vi "File Page - Set .NET Filter.vi"(7 "Include Wfms?":bool, 8 "error in (no error)":errorcluster, 11 "Trigger Control in":T1) -> (0 "error out":errorcluster, 3 "Trigger Control out":T1)   [LabVIEW 2015, in "Waveform Data Logger System Explorer.lvlib"]
uses:
  Waveform Data Logger System Explorer.lvlib
  <vilib>/NI Veristand/UI Controls/Single Node Browser/Single Node Browser Ref.ctl
  NationalInstruments.VeriStand.SystemStorageUI
  NationalInstruments.VeriStand.SystemStorage
  <vilib>/NI VeriStand/UI Controls/Single Node Browser/NI_VS UI Single Node Browser.lvlib
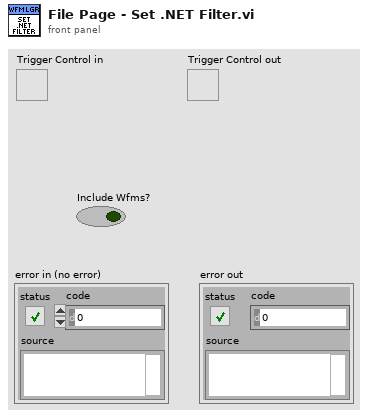
[diagram p1: front panel]
types:
  T1 = typedef "NI_VS UI Single Node Browser.lvlib/Single Node Browser Ref.ctl" = refnum<k24>
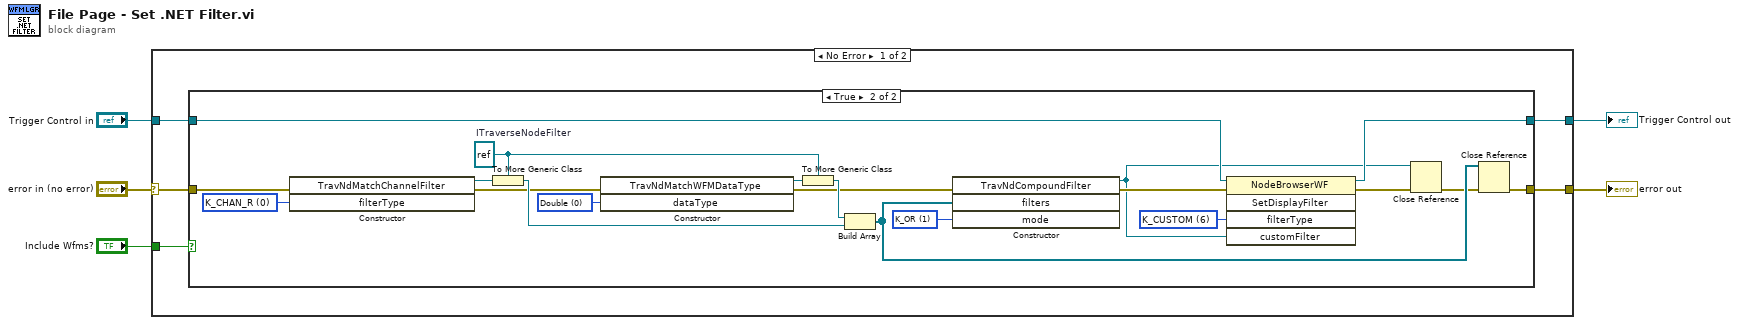
[diagram p0: block diagram]
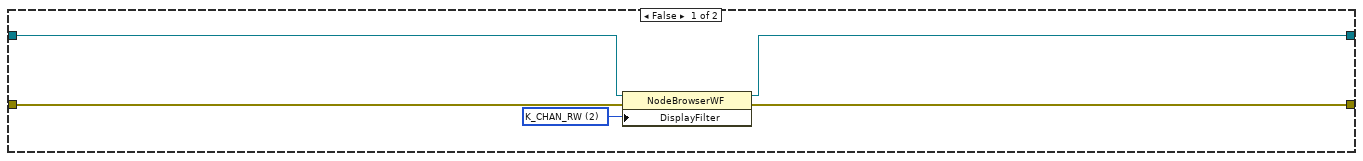
[diagram p2: hidden frame]
diagram:
  n1 = case shown="No Error" "error in (no error)" {
    selector: "error in (no error)" -> [w8 w37]
    tunnel: [w7 w37] -> w5
    tunnel: "Include Wfms?" -> [w10 _]
    tunnel: "Trigger Control in" -> [w9 w36]
    tunnel: [w6 w36] -> w2
    frame No Error {
      n2 = case shown="True" w10 {
        tunnel: w9 -> [w14 w26]
        tunnel: w8 -> [w13 w24]
        tunnel: [w12 w16] -> w7
        tunnel: [w11 w25] -> w6
        frame False {
          w15 = u8 2 items=["K_CHAN_R", "K_CHAN_W", "K_CHAN_RW", "K_CHAN_VOLT", "K_CHAN_FAULT", "K_ALL", "K_CUSTOM", "K_CHAN_R_VIS", "K_CHAN_W_VIS", "K_CHAN_RW_VIS", "K_CHAN_VOLT_VIS", "K_CHAN_FAULT_VIS", "K_WAVE", "K_WAVE_VIS", "K_WAVE_DBL", "K_WAVE_CDB", "K_WAVE_DBL_VIS", "K_WAVE_CDB_VIS"] ("DisplayFilter")
          n3 = property class="NodeBrowserWF"(reference=w14, error in=w13, "DisplayFilter"=w15) -> (reference out=w11:T1, error out=w12:errorcluster)
        }
        frame True {
          w28 = 0 items=["Double", "ComplexDouble"] ("dataType")
          w35 = u8 6 items=["K_CHAN_R", "K_CHAN_W", "K_CHAN_RW", "K_CHAN_VOLT", "K_CHAN_FAULT", "K_ALL", "K_CUSTOM", "K_CHAN_R_VIS", "K_CHAN_W_VIS", "K_CHAN_RW_VIS", "K_CHAN_VOLT_VIS", "K_CHAN_FAULT_VIS", "K_WAVE", "K_WAVE_VIS", "K_WAVE_DBL", "K_WAVE_CDB", "K_WAVE_DBL_VIS", "K_WAVE_CDB_VIS"] ("filterType")
          w27 = refnum<k24> refnum  # ITraverseNodeFilter
          w33 = 1 items=["K_AND", "K_OR"] ("mode")
          w34 = u8 0 items=["K_CHAN_R", "K_CHAN_W", "K_CHAN_VOLT", "K_CHAN_FAULT"] ("filterType")
          n4 = constructor class="TravNdMatchChannelFilter"(error in=w24, "filterType"=w34) -> (reference out=w32:refnum<k24>, error out=w23:errorcluster)  [unwired: 2 in, 2 out]
          n5 = To More Generic Class(target class=w27, reference=w32) -> (generic class reference=w31:refnum<k24>)
          n6 = constructor class="TravNdMatchWFMDataType"(error in=w23, "dataType"=w28) -> (reference out=w30:refnum<k24>, error out=w22:errorcluster)  [unwired: 2 in, 2 out]
          n7 = To More Generic Class(target class=w27, reference=w30) -> (generic class reference=w29:refnum<k24>)
          n8 = Build Array(w29, w31) -> (w18:refnum<k24>[])
          n9 = constructor class="TravNdCompoundFilter"(error in=w22, "filters"=w18, "mode"=w33) -> (reference out=w19:refnum<k24>, error out=w21:errorcluster)  [unwired: 2 in, 3 out]
          n10 = invoke class="NodeBrowserWF" method="SetDisplayFilter"(reference=w26, error in=w21, "filterType"=w35, "customFilter"=w19) -> (reference out=w25:T1, error out=w20:errorcluster)  [unwired: 1 in, 3 out]
          n11 = Close Reference(reference=w19, error in (no error)=w20) -> (error out=w17:errorcluster)
          n12 = Close Reference(reference=w18, error in (no error)=w17) -> (error out=w16:errorcluster)
        }
      }
    }
    frame Error {
    }
  }
  "error out" <- w5
  "Trigger Control out" <- w2
